vi "EndScript.vi"(8 "error in (no error)":errorcluster, 11 "Python":T1) -> (0 "error out":errorcluster, 2 "Tx for stopping code":string, 3 "Python":T1)   [LabVIEW 2020]
uses:
  PythonCtrl.ctl
  Processors.ctl
panel:
  out "Reply":string
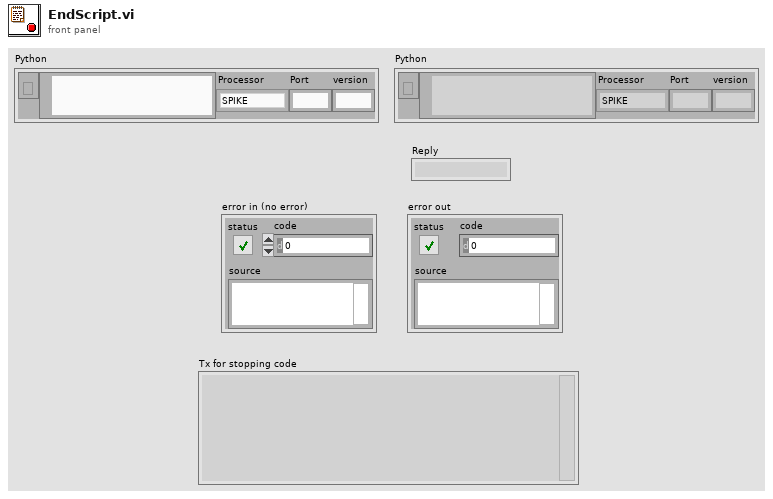
[diagram p1: front panel]
types:
  T1 = typedef "PythonCtrl.ctl" = cluster{"session":refnum<k35>, "PyPath":path, "Processor":T2, "Port":string, "version":string}
  T2 = typedef "Processors.ctl" = enum16{"SPIKE", "Pi", "Pi_ssh", "OpenMV", "Dunio"}
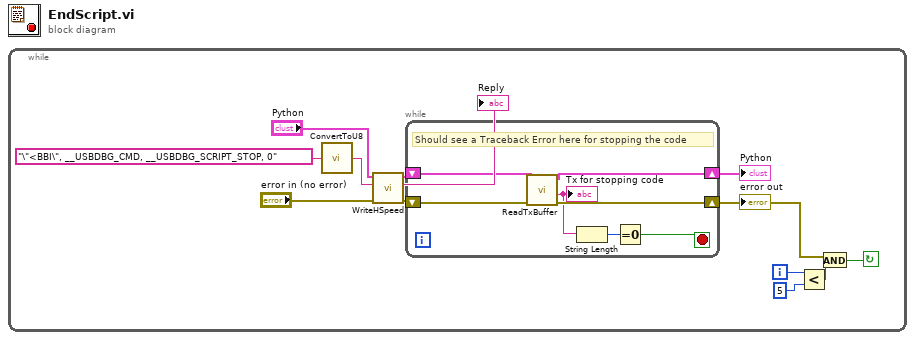
[diagram p0: block diagram]
diagram:
  n1 = while {
    i -> [w5]
    stop <- w1 continue-if-true
    n2 = call "ConvertToU8.vi"("struct"="\"<BBI\", __USBDBG_CMD, __USBDBG_SCRIPT_STOP, 0" ("write buffer")) -> ("Binary"=w9:string)
    n3 = call "WriteHSpeed.vi"("error in"="error in (no error)", "write buffer"=w9, "Python"="Python") -> ("error out"=w8:errorcluster, "read buffer"=→"Reply":string, "Python"=w7:T1)  [unwired: 6 in]
    n4 = while {
      shift-right: [w17] -> w2
      shift-left: w8 -> [w20]
      shift-right: [w18] -> w6
      shift-left: w7 -> [w19]
      stop <- w14 stop-if-true
      # "Should see a Traceback Error here for stopping the code"
      n5 = call "ReadTxBuffer.vi"("error in"=w20, "Python"=w19) -> ("error out"=w17:errorcluster, "Tx Buffer"=w16:string, "Python"=w18:T1)  [unwired: 6 in, 1 out]
      "Tx for stopping code" <- w16
      n6 = String Length(string=w16) -> (length=w15:i32)
      n7 = Equal To 0?(x=w15) -> (x = 0?=w14:bool)
    }
    "error out" <- w2
    "Python" <- w6
    n8 = Less?(x=w5, y=5) -> (x < y?=w3:bool)
    n9 = And(x=w2, y=w3) -> (x .and. y?=w1:bool)
  }
